vi "BitsToTemp.vi"(8 "Error In":errorcluster, 11 "Raw I2C Packets":u8[](array[numeric])) -> (0 "Error Out":errorcluster, 2 "Temperature (F)":dbl, 3 "Array":bool[](array[boolean]))   [LabVIEW 2015]
doc: "Takes raw packets of data from I2C sensor (MSB & LSB), combines, drops status bits, and coverts to raw temperature using formula in Page 15 of Data Sheet"
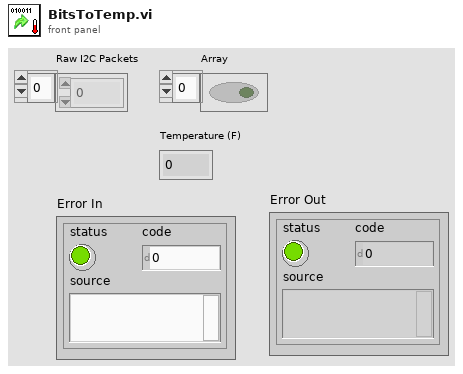
[diagram p1: front panel]
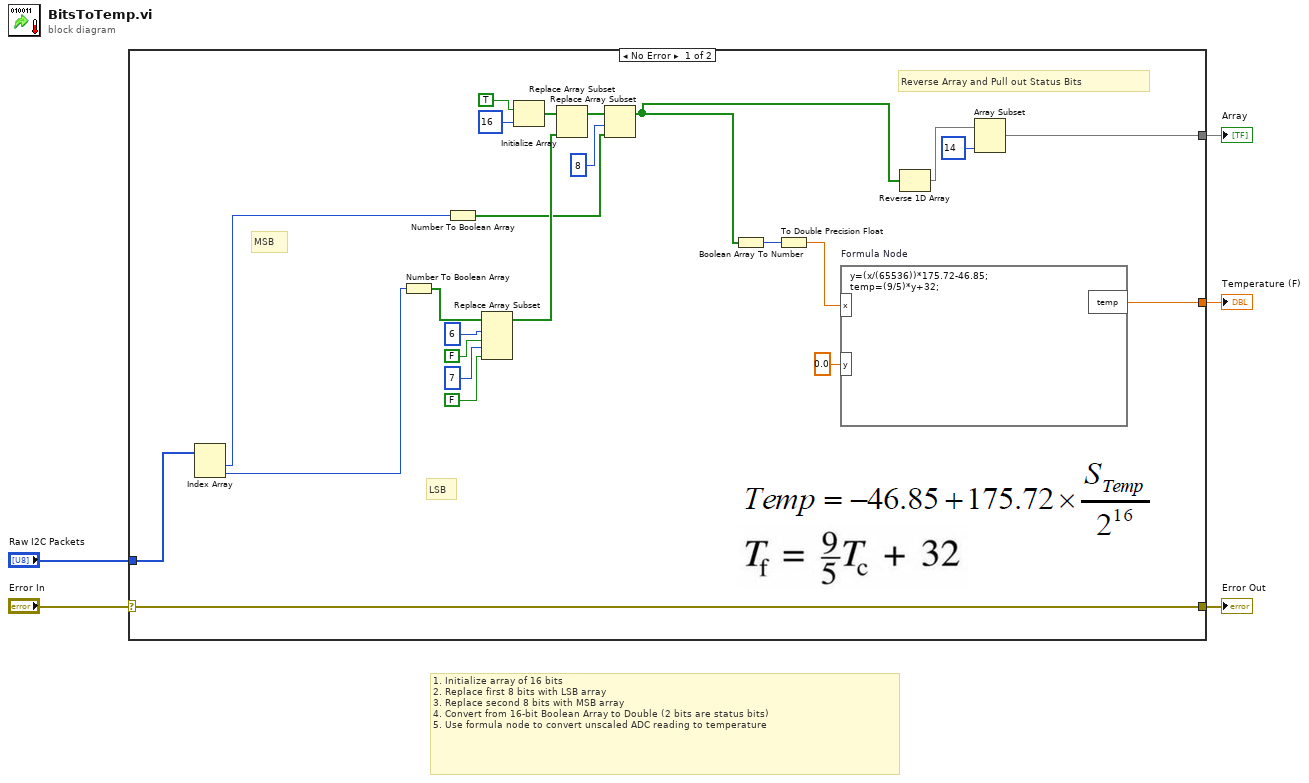
[diagram p0: block diagram]
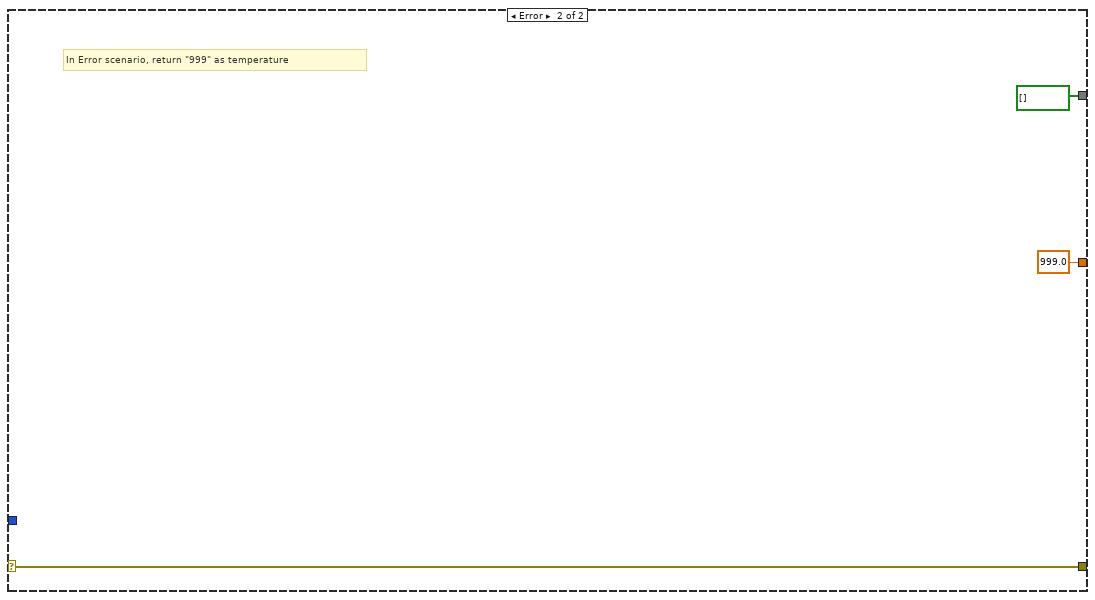
[diagram p2: hidden frame]
diagram:
  # "1. Initialize array of 16 bits\n2. Replace first 8 bits with LSB array\n3. Replace second 8 bits with MSB array\n4. Convert from 16-bit Boolean Array to Double (2 bits are status bits)\n5. Use formula node to convert unscaled ADC reading to temperature"
  n1 = case shown="No Error" "Error In" {
    selector: "Error In" -> [w6 w32]
    tunnel: [w12 999.0 ("temp")] -> w5
    tunnel: "Raw I2C Packets" -> [w11 _]
    tunnel: [w7 bool[] []] -> w3
    tunnel: [w6 w32] -> w1
    frame No Error {
      # "LSB"
      # "MSB"
      # "Reverse Array and Pull out Status Bits"
      n2 = Index Array(array=w11) -> (element #1=w21:u8, element #2=w20:u8)  [unwired: 2 in]
      n3 = Number To Boolean Array(number=w20) -> (Boolean array=w27:bool[])
      n4 = Number To Boolean Array(number=w21) -> (Boolean array=w28:bool[])
      n5 = Replace Array Subset(array=w27, new element #1=FALSE ("new element/subarray"), index #1=6 ("index"), new element #2=FALSE ("new element/subarray"), index #2=7 ("index")) -> (w29:bool[])
      n6 = Initialize Array(TRUE, 16 ("dimension size")) -> (w24:bool[])
      n7 = Replace Array Subset(array=w24, new element=w29) -> (w25:bool[])  [unwired: 1 in]
      n8 = Replace Array Subset(array=w25, new element=w28, index=8) -> (w8:bool[])
      n9 = Boolean Array To Number(Boolean array=w8) -> (number=w14:u32)
      n10 = To Double Precision Float(number=w14) -> (double precision float=w15:dbl)
      n11 = formula code="y=(x/(65536))*175.72-46.85; \ntemp=(9/5)*y+32;"("x"=w15, "y"=0.0 ("input variable")) -> ("temp"=w12:dbl)
      n12 = Reverse 1D Array(array=w8) -> (reversed array=w10:bool[])
      n13 = Array Subset(array=w10, length=14) -> (w7:bool[])  [unwired: 1 in]
    }
    frame Error {
      # "In Error scenario, return \"999\" as temperature"
    }
  }
  "Array" <- w3
  "Temperature (F)" <- w5
  "Error Out" <- w1
